vi "SParam Save S2P.vi"(8 "error in":errorcluster, 10 "Test Configuration":T1={"Action"=enum."Calibrate", "Power Level (dBm)"=0.0, "External Gain (dB)"=0.0, "Frequency Sweep"={"Start Frequency (Hz)"=4000000000.0, "Stop Frequency (Hz)"=26500000000.0, "Step Size (Hz)"=200.0}, "Type of Stimulus"=enum."CW", "Pulse Width (s)"=0.0, "PRI (s)"=0.0, "IF Bandwidth (Hz)"=0.0, "Average Mode"=enum."Per Sweep", "Number of Averages"=0, "SnP File Path"=path "", "Calibration File Path"=path ""} {"Frequency Sweep"."Step Size (Hz)" format="%#_6p"; "Frequency Sweep"."Stop Frequency (Hz)" format="%.3p"; "Frequency Sweep"."Start Frequency (Hz)" format="%.3p"}, 11 "S-Par Reference In":T2) -> (0 "error out":errorcluster, 3 "S-Par Reference Out":T2)   [LabVIEW 2023]
uses:
  <vilib>/niSPML/Typedefs/Session Handle.ctl
  <vilib>/niSPML/S-Par Reference.lvclass
  Controls/Test Config - SParam_VST.ctl
  <vilib>/niSPML/S-Parameter Measurements.lvlib
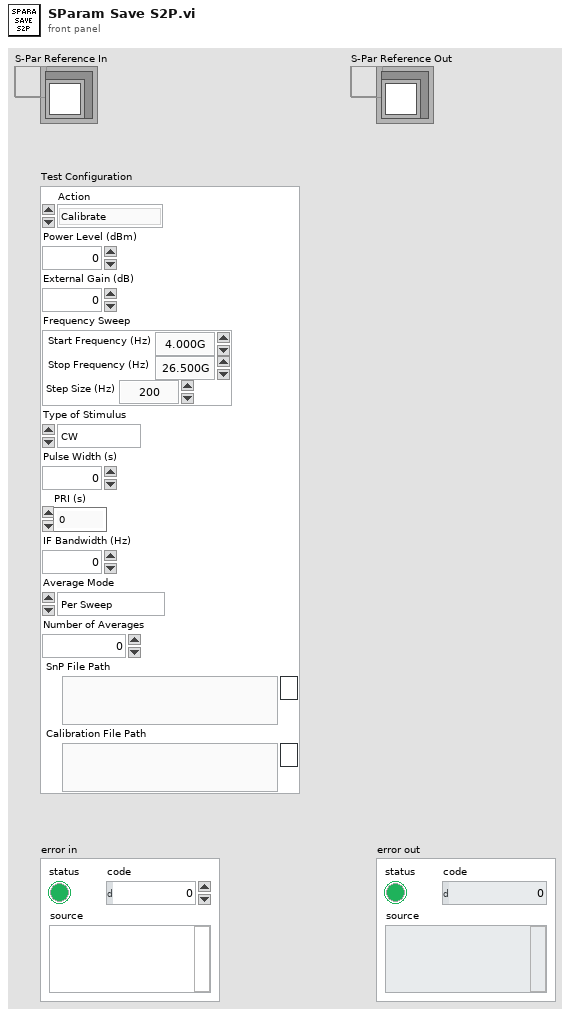
[diagram p1: front panel]
types:
  T1 = typedef "Test Config - SParam_VST.ctl" = cluster{"Action":enum32{"Calibrate", "Measure"}, "Power Level (dBm)":dbl, "External Gain (dB)":dbl, "Frequency Sweep":cluster{"Start Frequency (Hz)":dbl, "Stop Frequency (Hz)":dbl, "Step Size (Hz)":dbl}, "Type of Stimulus":enum16{"CW", "Pulsed CW"}, "Pulse Width (s)":dbl, "PRI (s)":dbl, "IF Bandwidth (Hz)":dbl, "Average Mode":enum16{"Per Sweep", "Per Point"}, "Number of Averages":i32, "SnP File Path":path, "Calibration File Path":path}
  T2 = typedef "S-Parameter Measurements.lvlib/S-Par Reference.lvclass/Session Handle.ctl" = refnum<data-value>
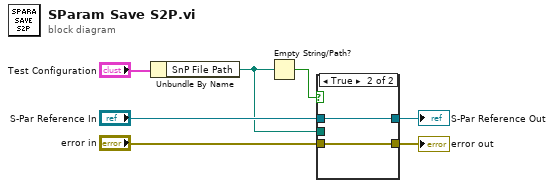
[diagram p0: block diagram]
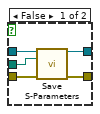
[diagram p2: hidden frame]
diagram:
  n1 = Unbundle By Name("Test Configuration") -> ("SnP File Path"=w1:path)
  n2 = Empty String/Path?(string/path=w1) -> (empty?=w7:bool)
  n3 = case shown="True" w7 {
    tunnel: [w11 w13] -> w6
    tunnel: "error in" -> [w12 w13]
    tunnel: w1 -> [w10 _]
    tunnel: "S-Par Reference In" -> [w9 w14]
    tunnel: [w8 w14] -> w3
    frame False {
      n4 = call <vilib>:"Save S-Parameters.vi"("S-Par Reference In"=w9, "S-Parameters File Path"=w10, "error in"=w12) -> ("S-Par Reference Out"=w8:T2, "error out"=w11:errorcluster)  [unwired: 11 in]
    }
    frame True {
    }
  }
  "error out" <- w6
  "S-Par Reference Out" <- w3
